vi "Make_Plots.vi"(1 "System Monitor Variables":T1, 2 "JT-Cluster":T2={"V2"=FALSE, "V5"=FALSE, "V1"=FALSE, "V9"=FALSE, "F"=FALSE, "C"=FALSE, "V4"=FALSE, "Dump"=0, "P3"=0.0, "P1"=0.0, "P2"=0.0, "P5"=0.0, "Box Temp"=0.0, "Pressure 1"=0, "Pressure 2"=0, "Pressure 3"=15, "Pressure 4"=13, "Setpoint"=0.0, "MC Heater Output"=0.0, "Still Heater Output"=0.0, "Sorb  Heater Output"=0.0, "Heater"=[], "Pressures"=[]} {"Pressure 4" items=["Time", "LI1CH1", "LI1CH2", "LI2CH1", "LI2CH2", "LI3CH1", "LI3CH2", "Field", "Temperature", "Temperature 2", "Temperatrue 3", "Nitrogen_Level", "Helium_Level", "Heater_LS370", "Sorb_Heater", "Still_Heater", "Capacity", "Loss", "Magnet_Temperature", "Lambda_Pressure", "Lambda_Needle_Valve", "LS370-CH1-T", "LS370-CH2-T", "LS370-CH3-T", "LS370-CH4-T", "LS370-TC-T", "LS370-CH1-R", "LS370-CH2-R", "LS370-CH3-R", "LS370-CH4-R", "LS370-TC-R", "LS372-CH1-T", "LS372-CH2-T", "LS372-CH3-T", "LS372-CH4-T", "LS372-CH5-T", "LS372-CH1-R", "LS372-CH2-R", "LS372-CH3-R", "LS372-CH4-R", "LS372-CH5-R", "Nada", "Keithley_Res", "Keithley_Current", "VTI_Heater", "VTI_Needle Valve", "LS340_Heater", "Keithley_6221_Amplitude", "Keithley_6221_Frequency", "Condense_Pressure", "Still_Pressure", "FP_Out_Pressure", "Dump_Pressure", "V1", "V2", "V4", "V5", "V9", "Forepump", "Compressor", "Keihtley_6221_Offset", "BoxTemp", "By", "Bz", "Phi", "heater-recond (%)", "Dewar Pressure "]; "Pressure 3" items=["Time", "LI1CH1", "LI1CH2", "LI2CH1", "LI2CH2", "LI3CH1", "LI3CH2", "Field", "Temperature", "Temperature 2", "Temperatrue 3", "Nitrogen_Level", "Helium_Level", "Heater_LS370", "Sorb_Heater", "Still_Heater", "Capacity", "Loss", "Magnet_Temperature", "Lambda_Pressure", "Lambda_Needle_Valve", "LS370-CH1-T", "LS370-CH2-T", "LS370-CH3-T", "LS370-CH4-T", "LS370-TC-T", "LS370-CH1-R", "LS370-CH2-R", "LS370-CH3-R", "LS370-CH4-R", "LS370-TC-R", "LS372-CH1-T", "LS372-CH2-T", "LS372-CH3-T", "LS372-CH4-T", "LS372-CH5-T", "LS372-CH1-R", "LS372-CH2-R", "LS372-CH3-R", "LS372-CH4-R", "LS372-CH5-R", "Nada", "Keithley_Res", "Keithley_Current", "VTI_Heater", "VTI_Needle Valve", "LS340_Heater", "Keithley_6221_Amplitude", "Keithley_6221_Frequency", "Condense_Pressure", "Still_Pressure", "FP_Out_Pressure", "Dump_Pressure", "V1", "V2", "V4", "V5", "V9", "Forepump", "Compressor", "Keihtley_6221_Offset", "BoxTemp", "By", "Bz", "Phi", "heater-recond (%)", "Dewar Pressure "]; "Pressure 2" items=["Time", "LI1CH1", "LI1CH2", "LI2CH1", "LI2CH2", "LI3CH1", "LI3CH2", "Field", "Temperature", "Temperature 2", "Temperatrue 3", "Nitrogen_Level", "Helium_Level", "Heater_LS370", "Sorb_Heater", "Still_Heater", "Capacity", "Loss", "Magnet_Temperature", "Lambda_Pressure", "Lambda_Needle_Valve", "LS370-CH1-T", "LS370-CH2-T", "LS370-CH3-T", "LS370-CH4-T", "LS370-TC-T", "LS370-CH1-R", "LS370-CH2-R", "LS370-CH3-R", "LS370-CH4-R", "LS370-TC-R", "LS372-CH1-T", "LS372-CH2-T", "LS372-CH3-T", "LS372-CH4-T", "LS372-CH5-T", "LS372-CH1-R", "LS372-CH2-R", "LS372-CH3-R", "LS372-CH4-R", "LS372-CH5-R", "Nada", "Keithley_Res", "Keithley_Current", "VTI_Heater", "VTI_Needle Valve", "LS340_Heater", "Keithley_6221_Amplitude", "Keithley_6221_Frequency", "Condense_Pressure", "Still_Pressure", "FP_Out_Pressure", "Dump_Pressure", "V1", "V2", "V4", "V5", "V9", "Forepump", "Compressor", "Keihtley_6221_Offset", "BoxTemp", "By", "Bz", "Phi", "heater-recond (%)", "Dewar Pressure "]; "Pressure 1" items=["Time", "LI1CH1", "LI1CH2", "LI2CH1", "LI2CH2", "LI3CH1", "LI3CH2", "Field", "Temperature", "Temperature 2", "Temperatrue 3", "Nitrogen_Level", "Helium_Level", "Heater_LS370", "Sorb_Heater", "Still_Heater", "Capacity", "Loss", "Magnet_Temperature", "Lambda_Pressure", "Lambda_Needle_Valve", "LS370-CH1-T", "LS370-CH2-T", "LS370-CH3-T", "LS370-CH4-T", "LS370-TC-T", "LS370-CH1-R", "LS370-CH2-R", "LS370-CH3-R", "LS370-CH4-R", "LS370-TC-R", "LS372-CH1-T", "LS372-CH2-T", "LS372-CH3-T", "LS372-CH4-T", "LS372-CH5-T", "LS372-CH1-R", "LS372-CH2-R", "LS372-CH3-R", "LS372-CH4-R", "LS372-CH5-R", "Nada", "Keithley_Res", "Keithley_Current", "VTI_Heater", "VTI_Needle Valve", "LS340_Heater", "Keithley_6221_Amplitude", "Keithley_6221_Frequency", "Condense_Pressure", "Still_Pressure", "FP_Out_Pressure", "Dump_Pressure", "V1", "V2", "V4", "V5", "V9", "Forepump", "Compressor", "Keihtley_6221_Offset", "BoxTemp", "By", "Bz", "Phi", "heater-recond (%)", "Dewar Pressure "]; "Dump" scale=0.0..100.0}, 3 "Measurement Time (s)":dbl format="%#_13g", 4 "X-Axis (S)":i32) -> (0 "JT-Cluster 2":T2={"V2"=FALSE, "V5"=FALSE, "V1"=FALSE, "V9"=FALSE, "F"=FALSE, "C"=FALSE, "V4"=FALSE, "Dump"=0, "P3"=0.0, "P1"=0.0, "P2"=0.0, "P5"=0.0, "Box Temp"=0.0, "Pressure 1"=0, "Pressure 2"=0, "Pressure 3"=15, "Pressure 4"=0, "Setpoint"=0.0, "MC Heater Output"=0.0, "Still Heater Output"=0.0, "Sorb  Heater Output"=0.0, "Heater"=[], "Pressures"=[]} {"Pressure 4" items=["Time", "LI1CH1", "LI1CH2", "LI2CH1", "LI2CH2", "LI3CH1", "LI3CH2", "Field", "Temperature", "Temperature 2", "Temperatrue 3", "Nitrogen_Level", "Helium_Level", "Heater_LS370", "Sorb_Heater", "Still_Heater", "Capacity", "Loss", "Magnet_Temperature", "Lambda_Pressure", "Lambda_Needle_Valve", "LS370-CH1-T", "LS370-CH2-T", "LS370-CH3-T", "LS370-CH4-T", "LS370-TC-T", "LS370-CH1-R", "LS370-CH2-R", "LS370-CH3-R", "LS370-CH4-R", "LS370-TC-R", "LS372-CH1-T", "LS372-CH2-T", "LS372-CH3-T", "LS372-CH4-T", "LS372-CH5-T", "LS372-CH1-R", "LS372-CH2-R", "LS372-CH3-R", "LS372-CH4-R", "LS372-CH5-R", "Nada", "Keithley_Res", "Keithley_Current", "VTI_Heater", "VTI_Needle Valve", "LS340_Heater", "Keithley_6221_Amplitude", "Keithley_6221_Frequency", "Condense_Pressure", "Still_Pressure", "FP_Out_Pressure", "Dump_Pressure", "V1", "V2", "V4", "V5", "V9", "Forepump", "Compressor", "Keihtley_6221_Offset", "BoxTemp", "By", "Bz", "Phi", "heater-recond (%)", "Dewar Pressure "]; "Pressure 3" items=["Time", "LI1CH1", "LI1CH2", "LI2CH1", "LI2CH2", "LI3CH1", "LI3CH2", "Field", "Temperature", "Temperature 2", "Temperatrue 3", "Nitrogen_Level", "Helium_Level", "Heater_LS370", "Sorb_Heater", "Still_Heater", "Capacity", "Loss", "Magnet_Temperature", "Lambda_Pressure", "Lambda_Needle_Valve", "LS370-CH1-T", "LS370-CH2-T", "LS370-CH3-T", "LS370-CH4-T", "LS370-TC-T", "LS370-CH1-R", "LS370-CH2-R", "LS370-CH3-R", "LS370-CH4-R", "LS370-TC-R", "LS372-CH1-T", "LS372-CH2-T", "LS372-CH3-T", "LS372-CH4-T", "LS372-CH5-T", "LS372-CH1-R", "LS372-CH2-R", "LS372-CH3-R", "LS372-CH4-R", "LS372-CH5-R", "Nada", "Keithley_Res", "Keithley_Current", "VTI_Heater", "VTI_Needle Valve", "LS340_Heater", "Keithley_6221_Amplitude", "Keithley_6221_Frequency", "Condense_Pressure", "Still_Pressure", "FP_Out_Pressure", "Dump_Pressure", "V1", "V2", "V4", "V5", "V9", "Forepump", "Compressor", "Keihtley_6221_Offset", "BoxTemp", "By", "Bz", "Phi", "heater-recond (%)", "Dewar Pressure "]; "Pressure 2" items=["Time", "LI1CH1", "LI1CH2", "LI2CH1", "LI2CH2", "LI3CH1", "LI3CH2", "Field", "Temperature", "Temperature 2", "Temperatrue 3", "Nitrogen_Level", "Helium_Level", "Heater_LS370", "Sorb_Heater", "Still_Heater", "Capacity", "Loss", "Magnet_Temperature", "Lambda_Pressure", "Lambda_Needle_Valve", "LS370-CH1-T", "LS370-CH2-T", "LS370-CH3-T", "LS370-CH4-T", "LS370-TC-T", "LS370-CH1-R", "LS370-CH2-R", "LS370-CH3-R", "LS370-CH4-R", "LS370-TC-R", "LS372-CH1-T", "LS372-CH2-T", "LS372-CH3-T", "LS372-CH4-T", "LS372-CH5-T", "LS372-CH1-R", "LS372-CH2-R", "LS372-CH3-R", "LS372-CH4-R", "LS372-CH5-R", "Nada", "Keithley_Res", "Keithley_Current", "VTI_Heater", "VTI_Needle Valve", "LS340_Heater", "Keithley_6221_Amplitude", "Keithley_6221_Frequency", "Condense_Pressure", "Still_Pressure", "FP_Out_Pressure", "Dump_Pressure", "V1", "V2", "V4", "V5", "V9", "Forepump", "Compressor", "Keihtley_6221_Offset", "BoxTemp", "By", "Bz", "Phi", "heater-recond (%)", "Dewar Pressure "]; "Pressure 1" items=["Time", "LI1CH1", "LI1CH2", "LI2CH1", "LI2CH2", "LI3CH1", "LI3CH2", "Field", "Temperature", "Temperature 2", "Temperatrue 3", "Nitrogen_Level", "Helium_Level", "Heater_LS370", "Sorb_Heater", "Still_Heater", "Capacity", "Loss", "Magnet_Temperature", "Lambda_Pressure", "Lambda_Needle_Valve", "LS370-CH1-T", "LS370-CH2-T", "LS370-CH3-T", "LS370-CH4-T", "LS370-TC-T", "LS370-CH1-R", "LS370-CH2-R", "LS370-CH3-R", "LS370-CH4-R", "LS370-TC-R", "LS372-CH1-T", "LS372-CH2-T", "LS372-CH3-T", "LS372-CH4-T", "LS372-CH5-T", "LS372-CH1-R", "LS372-CH2-R", "LS372-CH3-R", "LS372-CH4-R", "LS372-CH5-R", "Nada", "Keithley_Res", "Keithley_Current", "VTI_Heater", "VTI_Needle Valve", "LS340_Heater", "Keithley_6221_Amplitude", "Keithley_6221_Frequency", "Condense_Pressure", "Still_Pressure", "FP_Out_Pressure", "Dump_Pressure", "V1", "V2", "V4", "V5", "V9", "Forepump", "Compressor", "Keihtley_6221_Offset", "BoxTemp", "By", "Bz", "Phi", "heater-recond (%)", "Dewar Pressure "]; "Dump" scale=0.0..100.0})   [LabVIEW 2016]
uses:
  JT-Status.ctl
  Global/Global Variables/System Monitor Cluster.ctl
panel:
  # "Dill. unit"
  # "LN2\nTrap"
  # "12"
  # "15"
  # "Dill. unit"
  # "LN2\nTrap"
  # "12"
  # "15"
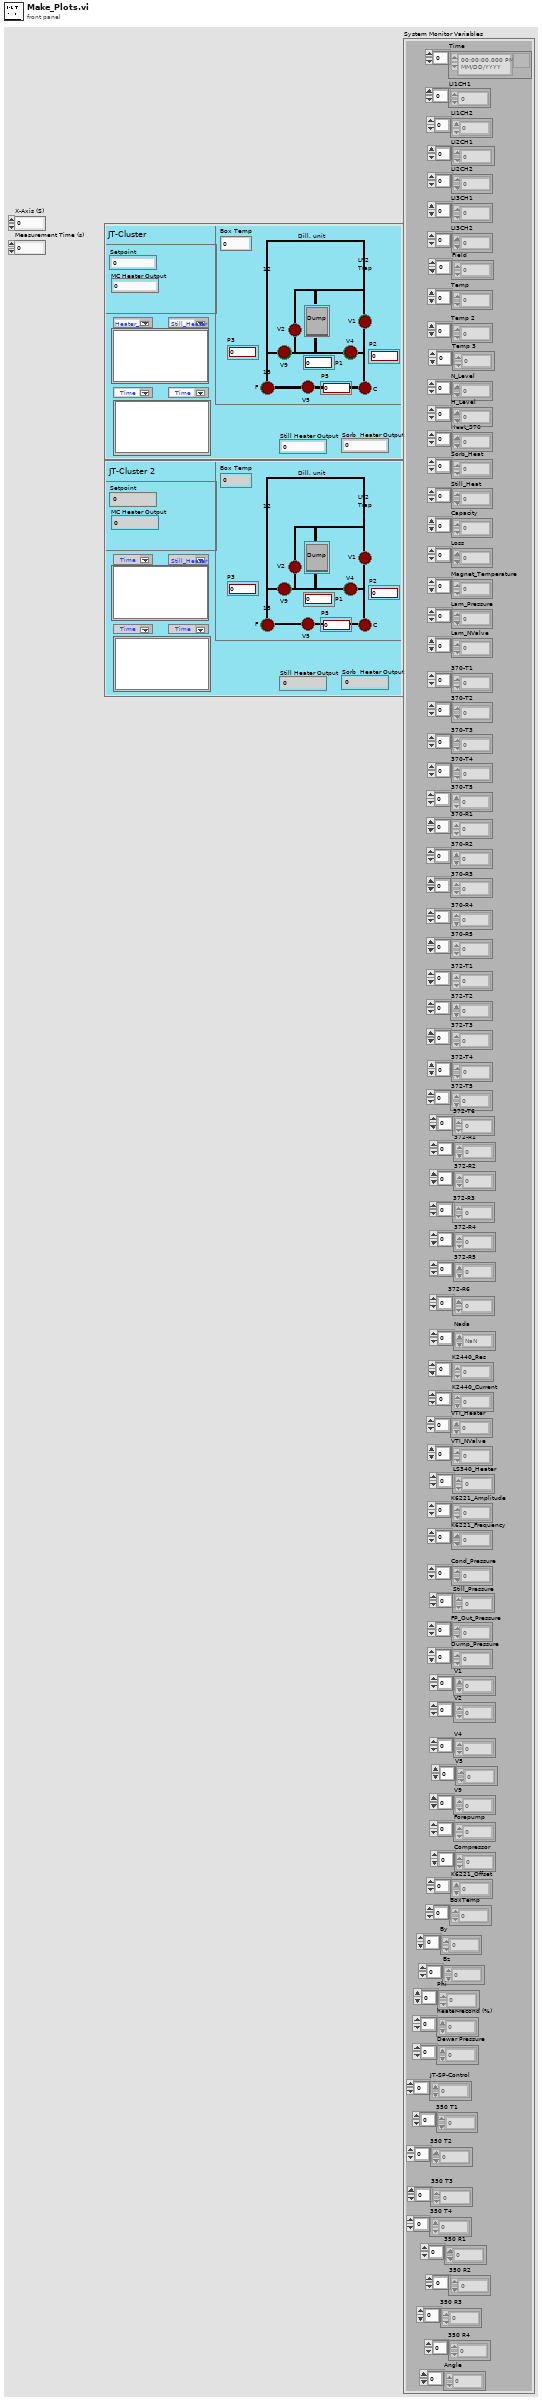
[diagram p1: front panel]
types:
  T1 = typedef "System Monitor Cluster.ctl" = cluster{"Time":timestamp[], "LI1CH1":dbl[], "LI1CH2":dbl[], "LI2CH1":dbl[], "LI2CH2":dbl[], "LI3CH1":dbl[], "LI3CH2":dbl[], "Field":dbl[], "Temp":dbl[], "Temp 2":dbl[], "Temp 3":dbl[], "N_Level":dbl[], "H_Level":dbl[], "Heat_370":dbl[], "Sorb_Heat":dbl[], "Still_Heat":dbl[], "Capacity":dbl[], "Loss":dbl[], "Magnet_Temperature":dbl[], "Lam_Pressure":dbl[], "Lam_NValve":dbl[], "370-T1":dbl[], "370-T2":dbl[], "370-T3":dbl[], "370-T4":dbl[], "370-T5":dbl[], "370-R1":dbl[], "370-R2":dbl[], "370-R3":dbl[], "370-R4":dbl[], "370-R5":dbl[], "372-T1":dbl[], "372-T2":dbl[], "372-T3":dbl[], "372-T4":dbl[], "372-T5":dbl[], "372-T6":dbl[], "372-R1":dbl[], "372-R2":dbl[], "372-R3":dbl[], "372-R4":dbl[], "372-R5":dbl[], "372-R6":dbl[], "Nada":dbl[], "K2440_Res":dbl[], "K2440_Current":dbl[], "VTI_Heater":dbl[], "VTI_NValve":dbl[], "LS340_Heater":dbl[], "K6221_Amplitude":dbl[], "K6221_Frequency":dbl[], "Cond_Pressure":dbl[], "Still_Pressure":dbl[], "FP_Out_Pressure":dbl[], "Dump_Pressure":dbl[], "V1":dbl[], "V2":dbl[], "V4":dbl[], "V5":dbl[], "V9":dbl[], "Forepump":dbl[], "Compressor":dbl[], "K6221_Offset":dbl[], "BoxTemp":dbl[], "By":dbl[], "Bz":dbl[], "Phi":dbl[], "heater-recond (%)":dbl[], "Dewar Pressure ":dbl[], "JT-SP-Control":dbl[], "350 T1":dbl[], "350 T2":dbl[], "350 T3":dbl[], "350 T4":dbl[], "350 R1":dbl[], "350 R2":dbl[], "350 R3":dbl[], "350 R4":dbl[], "Angle":dbl[]}
  T2 = typedef "JT-Status.ctl" = cluster{"V2":bool, "V5":bool, "V1":bool, "V9":bool, "F":bool, "C":bool, "V4":bool, "Dump":u8, "P3":dbl, "P1":dbl, "P2":dbl, "P5":dbl, "Box Temp":dbl, "Pressure 1":i16, "Pressure 2":i16, "Pressure 3":i16, "Pressure 4":i16, "Setpoint":dbl, "MC Heater Output":dbl, "Still Heater Output":dbl, "Sorb  Heater Output":dbl, "Heater":dbl[][], "Pressures":dbl[][]}
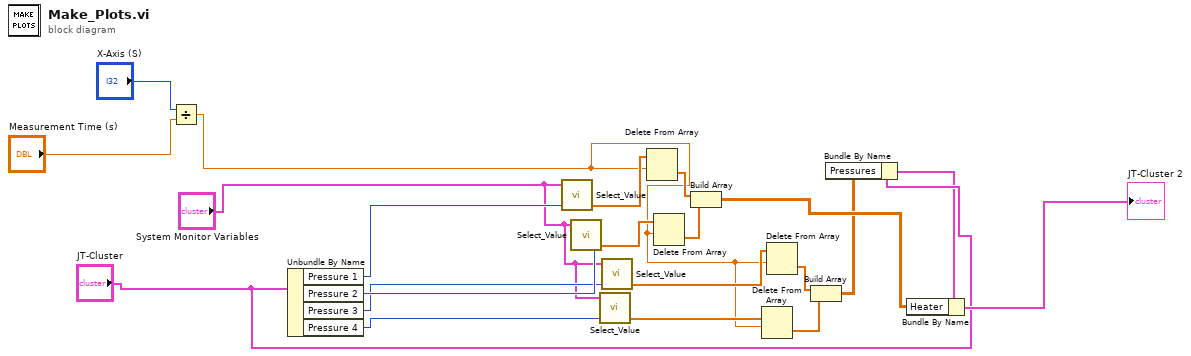
[diagram p0: block diagram]
diagram:
  n1 = Divide(x="X-Axis (S)", y="Measurement Time (s)") -> (x/y=w6:dbl)
  n2 = Unbundle By Name("JT-Cluster") -> ("Pressure 1"=w17:i16, "Pressure 2"=w16:i16, "Pressure 3"=w15:i16, "Pressure 4"=w14:i16)
  n3 = call "Select_Value.vi"("Numerisch"=w17, "System Monitor Variables"="System Monitor Variables") -> ("Array"=w9:dbl[])  [unwired: 1 in, 2 out]
  n4 = call "Select_Value.vi"("Numerisch"=w16, "System Monitor Variables"="System Monitor Variables") -> ("Array"=w10:dbl[])  [unwired: 1 in, 2 out]
  n5 = call "Select_Value.vi"("Numerisch"=w14, "System Monitor Variables"="System Monitor Variables") -> ("Array"=w11:dbl[])  [unwired: 1 in, 2 out]
  n6 = call "Select_Value.vi"("Numerisch"=w15, "System Monitor Variables"="System Monitor Variables") -> ("Array"=w12:dbl[])  [unwired: 1 in, 2 out]
  n7 = Delete From Array(array=w9, length=w6) -> (deleted portion=w18:dbl[])  [unwired: 1 in, 1 out]
  n8 = Delete From Array(array=w10, length=w6) -> (deleted portion=w19:dbl[])  [unwired: 1 in, 1 out]
  n9 = Build Array(w18, w19) -> (w5:dbl[][])
  n10 = Delete From Array(array=w11, length=w6) -> (deleted portion=w21:dbl[])  [unwired: 1 in, 1 out]
  n11 = Delete From Array(array=w12, length=w6) -> (deleted portion=w20:dbl[])  [unwired: 1 in, 1 out]
  n12 = Build Array(w20, w21) -> (w2:dbl[][])
  n13 = Bundle By Name(cluster="JT-Cluster", "Pressures"=w2) -> (w3:T2)
  n14 = Bundle By Name(cluster=w3, "Heater"=w5) -> (→"JT-Cluster 2":T2)
